vi "deinitializeProgram.vi"   [LabVIEW 2015]
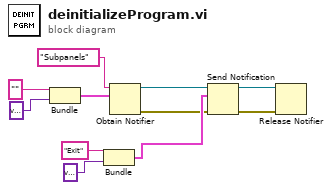
[diagram p0: block diagram]
diagram:
  n1 = Bundle("", variant) -> (w8:cluster{string, variant})  [unwired: 1 in]
  n2 = Bundle("Exit", variant) -> (w4:cluster{string, variant})  [unwired: 1 in]
  n3 = Obtain Notifier(name (unnamed)="Subpanels", notification data type=w8) -> (notifier out=w7:refnum<notifier>, error out=w1:errorcluster)  [unwired: 2 in, 1 out]
  n4 = Send Notification(notification=w4, notifier=w7, error in (no error)=w1) -> (notifier out=w3:refnum<notifier>, error out=w2:errorcluster)
  n5 = Release Notifier(notifier=w3, error in (no error)=w2) -> ()  [unwired: 1 in, 3 out]
